vi "Example Alarm.vi"() -> ()   [LabVIEW 2010]
uses:
  C:/tf/play/labview/Tinkerforge.dll
  Tinkerforge.dll
panel:
  in  "uid":string="amb"
  in  "port":i32=4223
  in  "host":string="localhost"
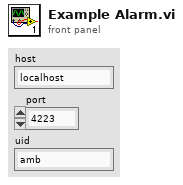
[diagram p1: front panel]
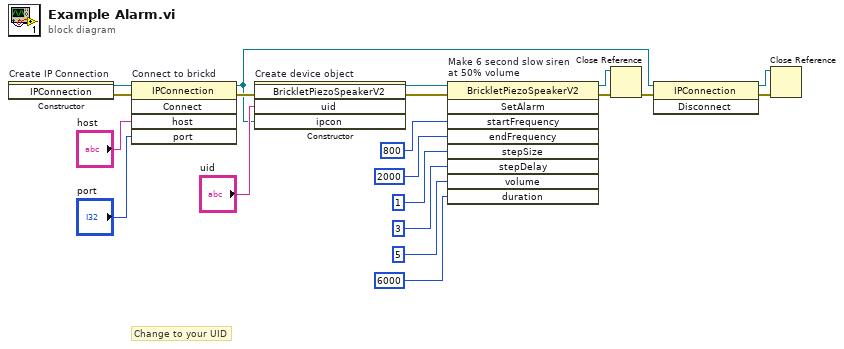
[diagram p0: block diagram]
diagram:
  # "Change to your UID"
  n1 = constructor on="Create IP Connection" class="IPConnection"() -> (reference out=w20:refnum<k24>, error out=w7:errorcluster)  [unwired: 3 in, 1 out]
  n2 = invoke on="Connect to brickd" class="IPConnection" method="Connect"(reference=w20, error in=w7, "host"="host", "port"="port") -> (reference out=w9:refnum<k24>, error out=w16:errorcluster)  [unwired: 1 in, 3 out]
  n3 = constructor on="Create device object" class="BrickletPiezoSpeakerV2"(error in=w16, "uid"="uid", "ipcon"=w9) -> (reference out=w14:refnum<k24>, error out=w15:errorcluster)  [unwired: 2 in, 3 out]
  n4 = invoke on="Make 6 second slow siren\nat 50% volume" class="BrickletPiezoSpeakerV2" method="SetAlarm"(reference=w14, error in=w15, "startFrequency"=800, "endFrequency"=2000, "stepSize"=1, "stepDelay"=3, "volume"=u8 5, "duration"=i64 6000) -> (reference out=w12:refnum<k24>, error out=w13:errorcluster)  [unwired: 1 in, 7 out]
  n5 = Close Reference(reference=w12, error in (no error)=w13) -> (error out=w11:errorcluster)
  n6 = invoke class="IPConnection" method="Disconnect"(reference=w9, error in=w11) -> (reference out=w8:refnum<k24>, error out=w10:errorcluster)  [unwired: 1 in, 1 out]
  n7 = Close Reference(reference=w8, error in (no error)=w10) -> ()  [unwired: 1 out]
